vi "Calculate_SNR_THD.vi"(0 "Auto Power Spectrum":dbl[](array[numeric]) format="%.4f", 1 "frame size":i32, 2 "# harmonics":i32=5 min=1 step=1, 3 "window":T1(ring), 4 "sampling rate":dbl=1.0 format="%.2f", 5 "fundamental frequency":dbl format="%.2f", 13 "integrate till":u16(ring) items=["Fs", "Fs/2", "Fs/4", "Fs/8", "Fs/16"], 16 "Blackman\n (fundamental power bins)":dbl=15.0 format="%.2f") -> (6 "% THD":dbl format="%.2f", 7 "ENOB(SNRD)":dbl format="%.2f", 8 "% THD + Noise":dbl format="%.2f", 9 "ENOB(SNR)":dbl format="%.2f", 10 "Noise Power":dbl format="%.2f", 11 "Fundamental frequency Calculated":dbl format="%.2f", 12 "SNR":dbl format="%.2f", 17 "Signal power":dbl format="%.2f", 18 "Harmonic Amplitudes":dbl[](array[numeric]) format="%.4f", 19 "Harmonic Frequencies":dbl[](array[numeric]) format="%.2f")   [LabVIEW 2021]
doc: "Finds the fundamental and harmonic components (amplitude and frequency) present in the input Auto Power Spectrum, and computes the %THD and the %THD plus noise.\n\nNOTE: You must pass the windowed auto power spectrum of your signal to this VI for it to function correctly. You should pass your time-domain signal through the Scaled Time Domain Window and then through the Auto Power Spectrum, connecting the Auto Power Spectrum to this VI.\n\nInputs\n-----------\nAuto Power Spectrum\n is the single-sided auto power spectrum of the windowed signal. This array can be the output of a frequency-domain averaging process for improved harmonic estimation.\n\nframe size\n is the number of samples in the original signal. Normally the frame size is the number of samples in one block of data from a data acquisition.\n\n# harmonics\n is the number of harmonic components that you want this VI to approximate and use in the harmonic analysis and THD measurement. This number includes the fundamental component. For example, if you wanted to compute the second harmonic distortion in your signal, this number should be two (find the fundamental frequency component (say, at f1 Hz) and its second harmonic (at f2 = 2f1 Hz).\n\nwindow\n is the window selection that you used for the Scaled Time Domain Window VI. If no window function was used (not recommended for an accurate THD estimation), this selector defaults to 0 (no window).\n\nsampling rate\n is the input sampling rate in Hz.\n\nfundamental frequency\n is an estimate of the fundamental frequency that you want this VI to use in the harmonic search and in the THD computation. If this control is set to zero (default), then the non-DC component with the maximum magnitude found in Auto Power Spectrum will be used as the fundamental component.\n\nOutputs\n-----------\nHarmonic Amplitudes\n is the array of amplitudes of the fundamental component and its harmonics. These values are always positive and are in units of Vrms if the input Auto Power Spectrum values are given in Vrms^2.\n\nHarmonic Frequencies\n is the array of frequencies of the fundamental component and its harmonics. These value are in units of Hz if the input sampling rate is given in Hz.\n\n% THD\n is the percent total harmonic distortion present in the input Auto Power Spectrum. The THD computation is computed using:\n\n % THD = 100 * sqrt[A(f2)^2 + A(f3)^2 + ... + A(fN^2)] / A(f1)\nwhere\n A(f1) is the amplitude of the fundamental component\n A(fN) is the amplitude of the Nth harmonic\n N is the # harmonics \n\n% THD + Noise\n is the percent total harmonic distortion plus noise present in the input Auto Power Spectrum. % THD + Noise is computed using:\n\n % THD + Noise = 100 * sqrt[sum(APS)] / A(f1)\nwhere\n sum(APS) is the sum of the Auto Power Spectrum without the power near DC and near the fundamental."
panel:
  out "FFT Magnitude Plot (dB)":dbl[](graph)
  # "Harmonic Analyzer"
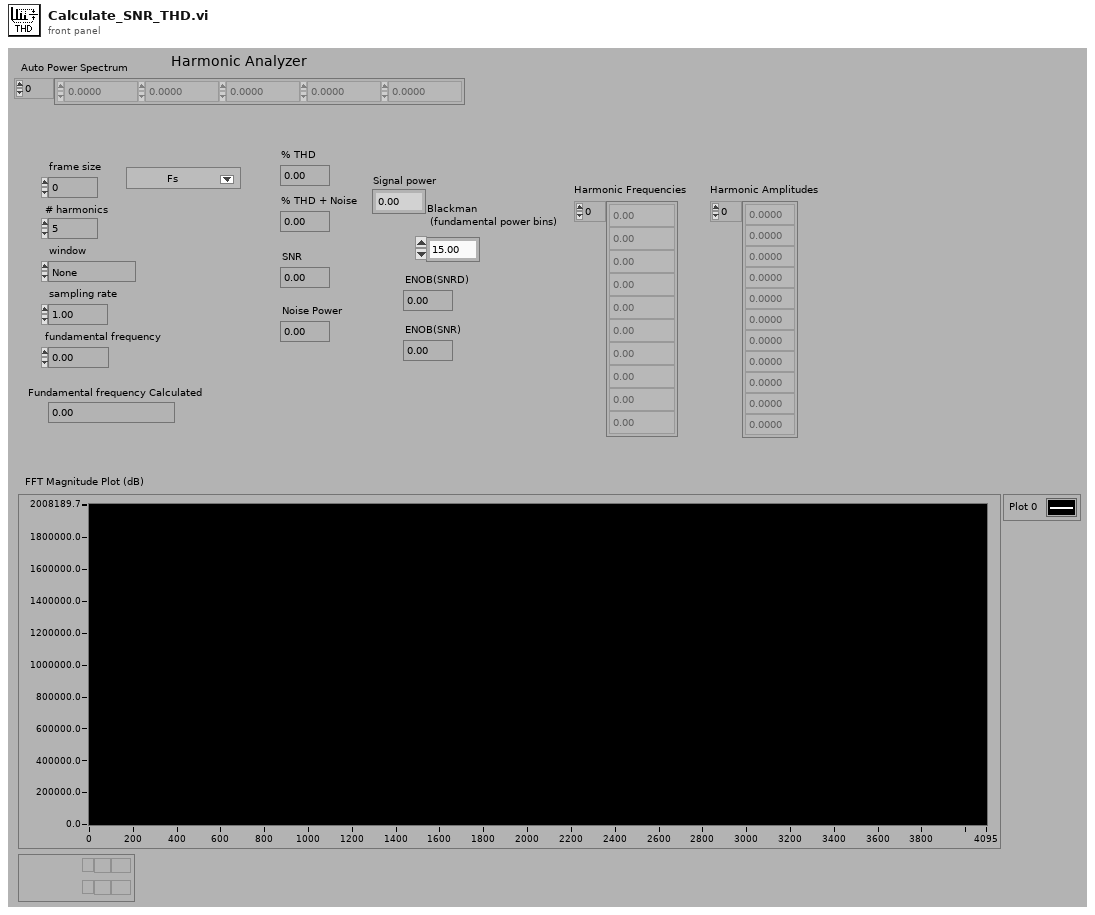
[diagram p1: front panel]
types:
  T1 = enum32{"None ", "Hanning", "Hamming", "Blackman-Harris", "Exact Blackman", "Blackman", "Flat Top", "4 Term B-Harris ", "7 Term B-Harris"}
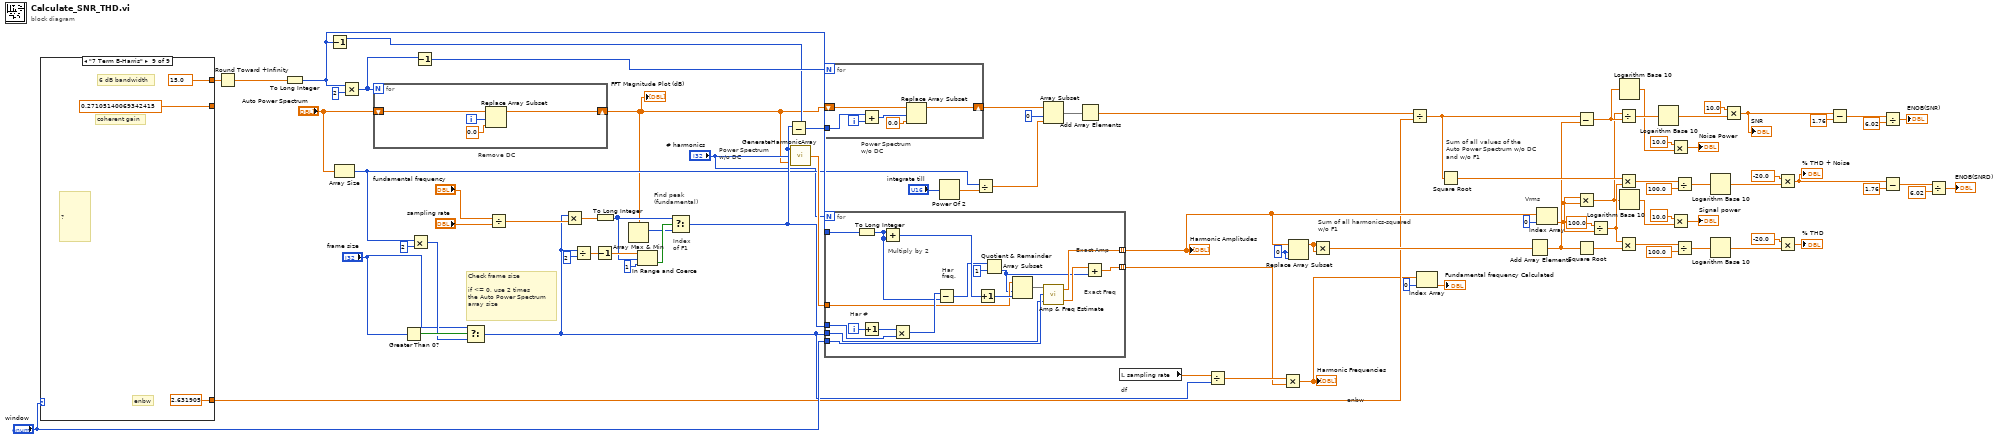
[diagram p0: block diagram]
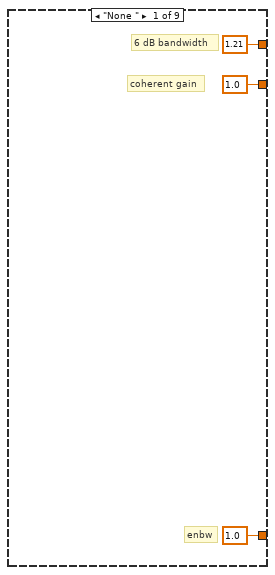
[diagram p2: hidden frame]
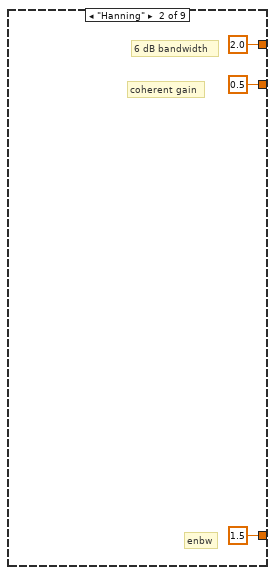
[diagram p3: hidden frame]
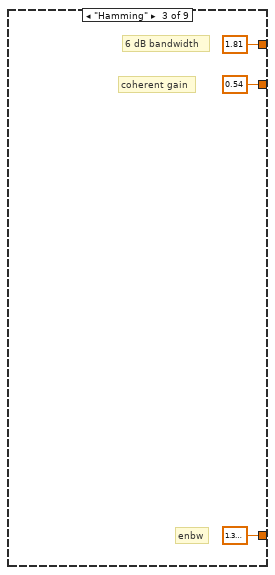
[diagram p4: hidden frame]
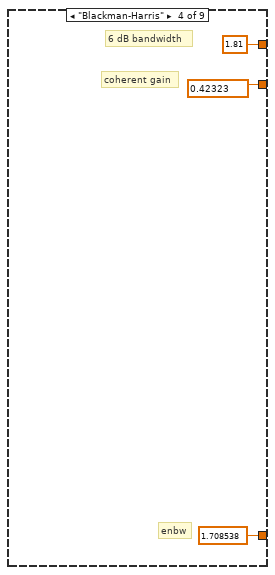
[diagram p5: hidden frame]
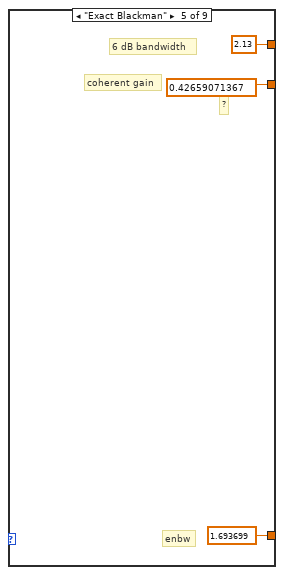
[diagram p6: hidden frame]
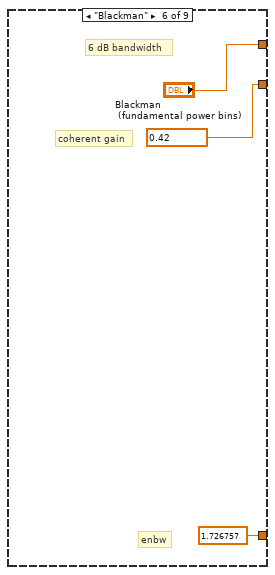
[diagram p7: hidden frame]
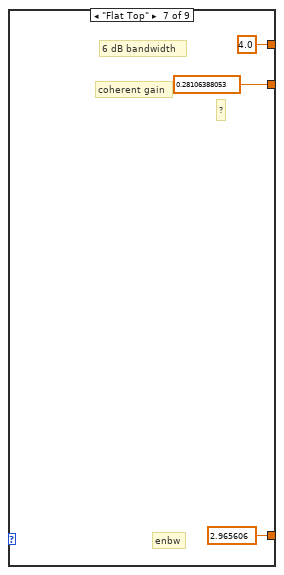
[diagram p8: hidden frame]
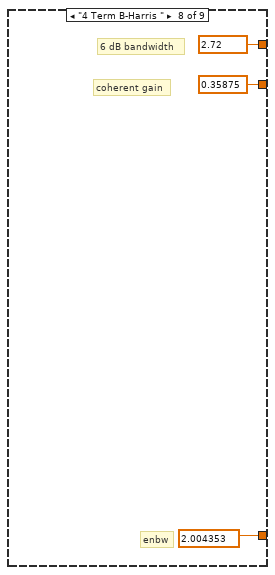
[diagram p9: hidden frame]
diagram:
  w86 = 0
  # "Check frame size\n\nif <= 0, use 2 times\nthe Auto Power Spectrum\narray size"
  # "enbw"
  # "df"
  # "Sum of all harmonics-squared\nw/o F1"
  # "Vrms"
  # "Sum of all values of the\nAuto Power Spectrum w/o DC\nand w/o F1"
  # "Power Spectrum\nw/o DC"
  # "Index \nof F1"
  # "Power Spectrum\nw/o DC"
  # "Find peak\n(fundamental)"
  # "Remove DC"
  n1 = case shown="\"7 Term B-Harris\"" "window" {
    tunnel: [1.0 0.5 0.54 0.42323 0.42659071367 0.42 0.28106388053 0.35875 0.27105140069342415] -> _
    tunnel: [1.0 1.5 1.362826 1.708538 1.693699 1.726757 2.965606 2.004353 2.631905] -> w61
    tunnel: [1.21 2.0 1.81 1.81 2.13 "Blackman\n (fundamental power bins)" 4.0 2.72 15.0] -> w60
    frame "None " {
      # "enbw"
      # "coherent gain"
      # "6 dB bandwidth"
    }
    frame "Hanning" {
      # "enbw"
      # "coherent gain"
      # "6 dB bandwidth"
    }
    frame "Hamming" {
      # "enbw"
      # "coherent gain"
      # "6 dB bandwidth"
    }
    frame "Blackman-Harris" {
      # "enbw"
      # "coherent gain"
      # "6 dB bandwidth"
    }
    frame "Exact Blackman" {
      # "enbw"
      # "coherent gain"
      # "6 dB bandwidth"
      # "?"
    }
    frame "Blackman" {
      # "enbw"
      # "coherent gain"
      # "6 dB bandwidth"
    }
    frame "Flat Top" {
      # "enbw"
      # "coherent gain"
      # "6 dB bandwidth"
      # "?"
    }
    frame "4 Term B-Harris " {
      # "enbw"
      # "coherent gain"
      # "6 dB bandwidth"
    }
    frame "7 Term B-Harris" {
      # "enbw"
      # "coherent gain"
      # "6 dB bandwidth"
      # "?"
    }
  }
  n2 = Round Toward +Infinity(x=w60) -> (ceil(x): smallest int >= x=w57:dbl)
  n3 = To Long Integer(number=w57) -> (32bit integer=w51:i32)
  n4 = Decrement(x=w51) -> (x-1=w82:i32)
  n5 = Array Size(array="Auto Power Spectrum") -> (size(s)=w10:i32)
  n6 = Multiply(x=w51, y=2) -> (x*y=w58:i32)
  n7 = for {
    N: w58 -> [_]
    shift-right: [w118] -> w1
    shift-left: "Auto Power Spectrum" -> [w117]
    i -> [w120]
    n8 = Replace Array Subset(array=w117, new element=0.0, index=w120) -> (w118:dbl[])
  }
  "FFT Magnitude Plot (dB)" <- w1
  n9 = Greater Than 0?(x="frame size") -> (x > 0?=w56:bool)
  n10 = Multiply(x=w10, y=2) -> (x*y=w54:i32)
  n11 = Decrement(x=w58) -> (x-1=w83:i32)
  n12 = Select(t="frame size", s=w56, f=w54) -> (s? t:f=w52:i32)
  n13 = Divide(x="fundamental frequency", y="sampling rate") -> (x/y=w66:dbl)
  n14 = Multiply(x=w52, y=w66) -> (x*y=w75:dbl)
  n15 = Divide(x=w52, y=2) -> (x/y=w77:dbl)
  n16 = To Long Integer(number=w75) -> (32bit integer=w73:i32)
  n17 = Decrement(x=w77) -> (x-1=w76:dbl)
  n18 = Array Max & Min(array=w1) -> (max index (indices)=w72:i32)  [unwired: 3 out]
  n19 = In Range and Coerce(upper limit=w76, x=w73, lower limit=1) -> (In Range?=w74:bool)  [unwired: 1 out]
  n20 = Select(t=w73, s=w74, f=w72) -> (s? t:f=w15:i32)
  n21 = Subtract(x=w15, y=w82) -> (x-y=w81:i32)
  n22 = call "GenerateHarmonicArray.vi"("Samples"=w1, "Harmonic"="# harmonics", "input"=w15) -> ("Ouput Samples"=w16:dbl[])
  n23 = for {
    N: w83 -> [_]
    shift-right: [w125] -> w11
    shift-left: w1 -> [w124]
    tunnel: w81 -> [w121]
    i -> [w123]
    n24 = Add(x=w121, y=w123) -> (x+y=w122:i32)
    n25 = Replace Array Subset(array=w124, new element=0.0, index=w122) -> (w125:dbl[])
  }
  n26 = for {
    N: "# harmonics" -> [_]
    tunnel: w16 -> [w140]
    tunnel: "window" -> [w138]
    tunnel: [w136] -> w67 mode=indexing
    tunnel: [w135] -> w68 mode=indexing
    tunnel: w15 -> [w129]
    tunnel: w52 -> [w128]
    tunnel: w51 -> [w127]
    i -> [w137]
    # "Multiply by 2"
    # "Exact Amp"
    # "Exact Freq"
    # "Har\nfreq."
    # "Har #"
    n27 = To Long Integer(number=w127) -> (32bit integer=w143:i32)
    n28 = Increment(x=w137) -> (x+1=w130:i32)
    n29 = Add(x=w143, y=w143) -> (x+y=w142:i32)
    n30 = Multiply(x=w130, y=w129) -> (x*y=w144:i32)
    n31 = Subtract(x=w144, y=w143) -> (x-y=w132:i32)
    n32 = Increment(x=w142) -> (x+1=w141:i32)
    n33 = Quotient & Remainder(x=w132, y=1) -> (floor(x/y)=w133:i32)  [unwired: 1 out]
    n34 = Array Subset(array=w140, index=w133, length=w141) -> (w139:dbl[])
    n35 = call "Amp & Freq Estimate.vi"("Size of FFT"=w128, "window"=w138, "Part of Power Spectrum"=w139) -> ("Exact Freq Index"=w134:dbl, "Exact Amplitude (Vrms)"=w136:dbl)
    n36 = Add(x=w134, y=w133) -> (x+y=w135:dbl)
  }
  "Harmonic Amplitudes" <- w67
  n37 = Power Of 2(x="integrate till") -> (2^x=w3:dbl)
  n38 = Divide(x=w10, y=w3) -> (x/y=w9:dbl)
  n39 = Array Subset(array=w11, index=0, length=w9) -> (w12:dbl[])
  n40 = Add Array Elements(numeric array=w12) -> (sum=w85:dbl)
  n41 = local read "sampling rate"() -> (w69:dbl)
  n42 = Divide(x=w69, y=w52) -> (x/y=w70:dbl)
  n43 = Multiply(x=w70, y=w68) -> (x*y=w28:dbl[])
  "Harmonic Frequencies" <- w28
  n44 = Replace Array Subset(array=w67, new element=w86, index=w86) -> (w2:dbl[])
  n45 = Multiply(x=w2, y=w2) -> (x*y=w87:dbl[])
  n46 = Divide(x=w85, y=w61) -> (x/y=w50:dbl)
  n47 = Index Array(array=w28, index=0) -> (element=→"Fundamental frequency Calculated":dbl)
  n48 = Square Root(x=w50) -> (sqrt(x)=w84:dbl)
  n49 = Add Array Elements(numeric array=w87) -> (sum=w49:dbl)
  n50 = Index Array(array=w67, index=0) -> (element=w48:dbl)
  n51 = Subtract(x=w50, y=w49) -> (x-y=w34:dbl)
  n52 = Multiply(x=w48, y=w48) -> (x*y=w6:dbl)
  n53 = Square Root(x=w49) -> (sqrt(x)=w63:dbl)
  n54 = Divide(x=100.0, y=w48) -> (x/y=w64:dbl)
  n55 = Divide(x=w6, y=w34) -> (x/y=w45:dbl)
  n56 = Multiply(x=w84, y=w64) -> (x*y=w29:dbl)
  n57 = Multiply(x=w64, y=w63) -> (x*y=w39:dbl)
  n58 = Logarithm Base 10(1:w34) -> (0:w37:dbl)
  n59 = Logarithm Base 10(1:w6) -> (0:w7:dbl)
  n60 = Logarithm Base 10(1:w45) -> (0:w47:dbl)
  n61 = Multiply(x=10.0, y=w37) -> (x*y=→"Noise Power":dbl)
  n62 = Multiply(x=10.0, y=w7) -> (x*y=→"Signal power":dbl)
  n63 = Divide(x=w29, y=100.0) -> (x/y=w32:dbl)
  n64 = Divide(x=w39, y=100.0) -> (x/y=w41:dbl)
  n65 = Logarithm Base 10(1:w32) -> (0:w31:dbl)
  n66 = Logarithm Base 10(1:w41) -> (0:w42:dbl)
  n67 = Multiply(x=10.0, y=w47) -> (x*y=w44:dbl)
  "SNR" <- w44
  n68 = Multiply(x=-20.0, y=w31) -> (x*y=w18:dbl)
  "% THD + Noise" <- w18
  n69 = Multiply(x=-20.0, y=w42) -> (x*y=→"% THD":dbl)
  n70 = Subtract(x=w44, y=1.76) -> (x-y=w24:dbl)
  n71 = Divide(x=w24, y=6.02) -> (x/y=→"ENOB(SNR)":dbl)
  n72 = Subtract(x=w18, y=1.76) -> (x-y=w20:dbl)
  n73 = Divide(x=w20, y=6.02) -> (x/y=→"ENOB(SNRD)":dbl)
